vi "Measurement Logic.vi"() -> ()   [LabVIEW 2024, in "OneShot-PureTone.lvlib"]
uses:
  OneShot-PureTone.lvlib
  <vilib>/Plug-In SDKs/Measurements/Measure Call Context/Measure Call Context.lvclass
  Measurement Configuration.ctl
  Measurement Results.ctl
  <vilib>/DAQmx/read.llb/DAQmx Read (Analog Wfm 1Chan NSamp).vi
  <vilib>/DAQmx/create/channels.llb/DAQmx Create Channel (AI-Voltage-Basic).vi
  <vilib>/DAQmx/configure/timing.llb/DAQmx Timing (Sample Clock).vi
  <vilib>/DAQmx/create/channels.llb/DAQmx Create Channel (AO-FuncGen).vi
  <vilib>/DAQmx/miscellaneous.llb/DAQmx Fill In Error Info.vi
  <extravilib>/ChannelInstances/Event Messenger-bool/Instantiate.vi
  <resource>/objmgr/daqmx.rc
panel:
  out "measurement results":T1={"band start (Hz) out"=0.0, "band stop (Hz) out"=0.0, "detected frequency (Hz)"=0.0, "detected amplitude"=0.0, "acquired response"=[0.0], "measurement subset"=[0.0], "acquired response t0"=0.0, "acquired response dt"=0.0, "measurement subset t0"=0.0, "measurement subset dt"=0.0, "THD maximum harmonic out"=9} {"THD maximum harmonic out" min=-1 max=1000; "detected amplitude" format="%.3g"; "band stop (Hz) out" format="%.2f"; "band start (Hz) out" format="%.2f"}
  in  "measurement configuration":T2={"THD maximum harmonic"=1, "measurement duration (s)"=1.2, "measurement cycles"=32.0, "band start (Hz)"=32.0, "band stop (Hz)"=64.0, "settle time (s)"=-32.0, "settle cycles"=-64.0, "AI range"=-64.0, "output channel"="Dev1/ao0", "input channel"="Dev1/ai0", "frequency (Hz)"=1.0, "amplitude"=1.0, "sample rate (Hz)"=0.05} {"sample rate (Hz)" min=0.0 format="%.2p"; "amplitude" format="%.3g"; "frequency (Hz)" format="±  %.3g"; "settle cycles" min=0.0 format="%.2p"; "band stop (Hz)" format="%.2f"; "measurement cycles" min=1.0; "THD maximum harmonic" min=-1 max=1000}
  out "measure call context out":refnum<class "Measure Call Context.lvclass">
  in  "measure call context in":refnum<class "Measure Call Context.lvclass">
  out "error out":errorcluster
  in  "error in":errorcluster
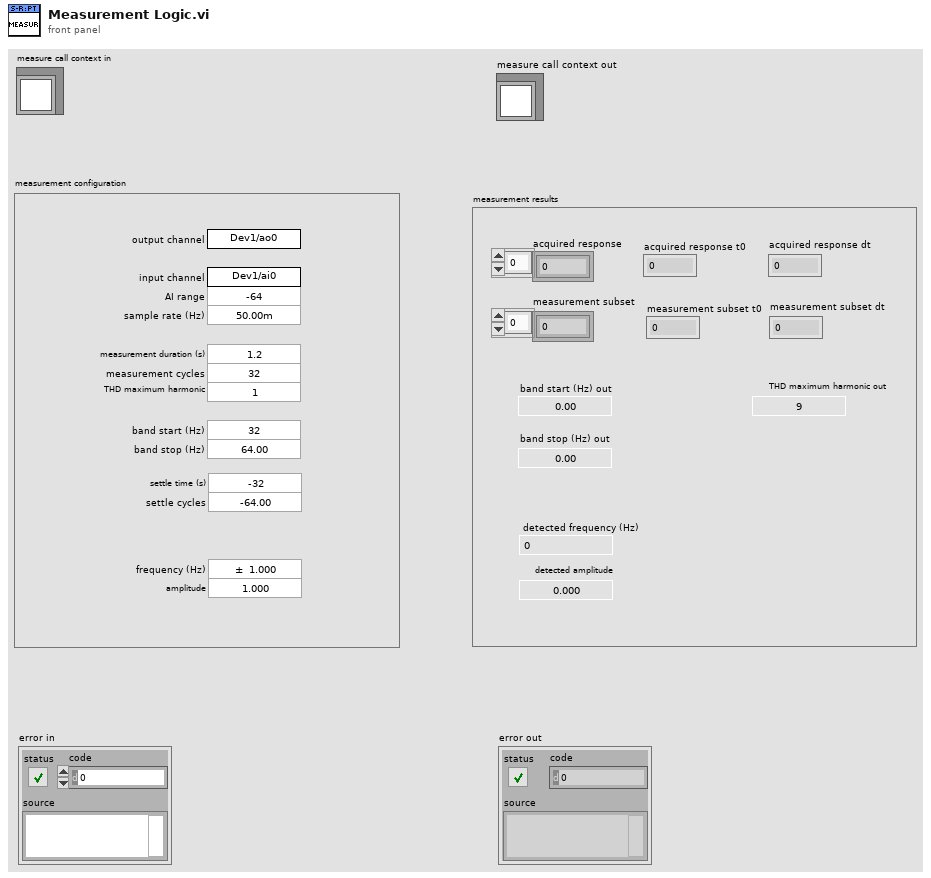
[diagram p1: front panel]
types:
  T1 = typedef "OneShot-PureTone.lvlib/Measurement Results.ctl" = cluster{"band start (Hz) out":dbl, "band stop (Hz) out":dbl, "detected frequency (Hz)":dbl, "detected amplitude":dbl, "acquired response":dbl[], "measurement subset":dbl[], "acquired response t0":dbl, "acquired response dt":dbl, "measurement subset t0":dbl, "measurement subset dt":dbl, "THD maximum harmonic out":i32}
  T2 = typedef "OneShot-PureTone.lvlib/Measurement Configuration.ctl" = cluster{"THD maximum harmonic":i32, "measurement duration (s)":dbl, "measurement cycles":dbl, "band start (Hz)":dbl, "band stop (Hz)":dbl, "settle time (s)":dbl, "settle cycles":dbl, "AI range":dbl, "output channel":string, "input channel":string, "frequency (Hz)":dbl, "amplitude":dbl, "sample rate (Hz)":dbl}
  T3 = typedef "Event Messenger-bool.lvlib/))Channel.ctl" = refnum<queue>
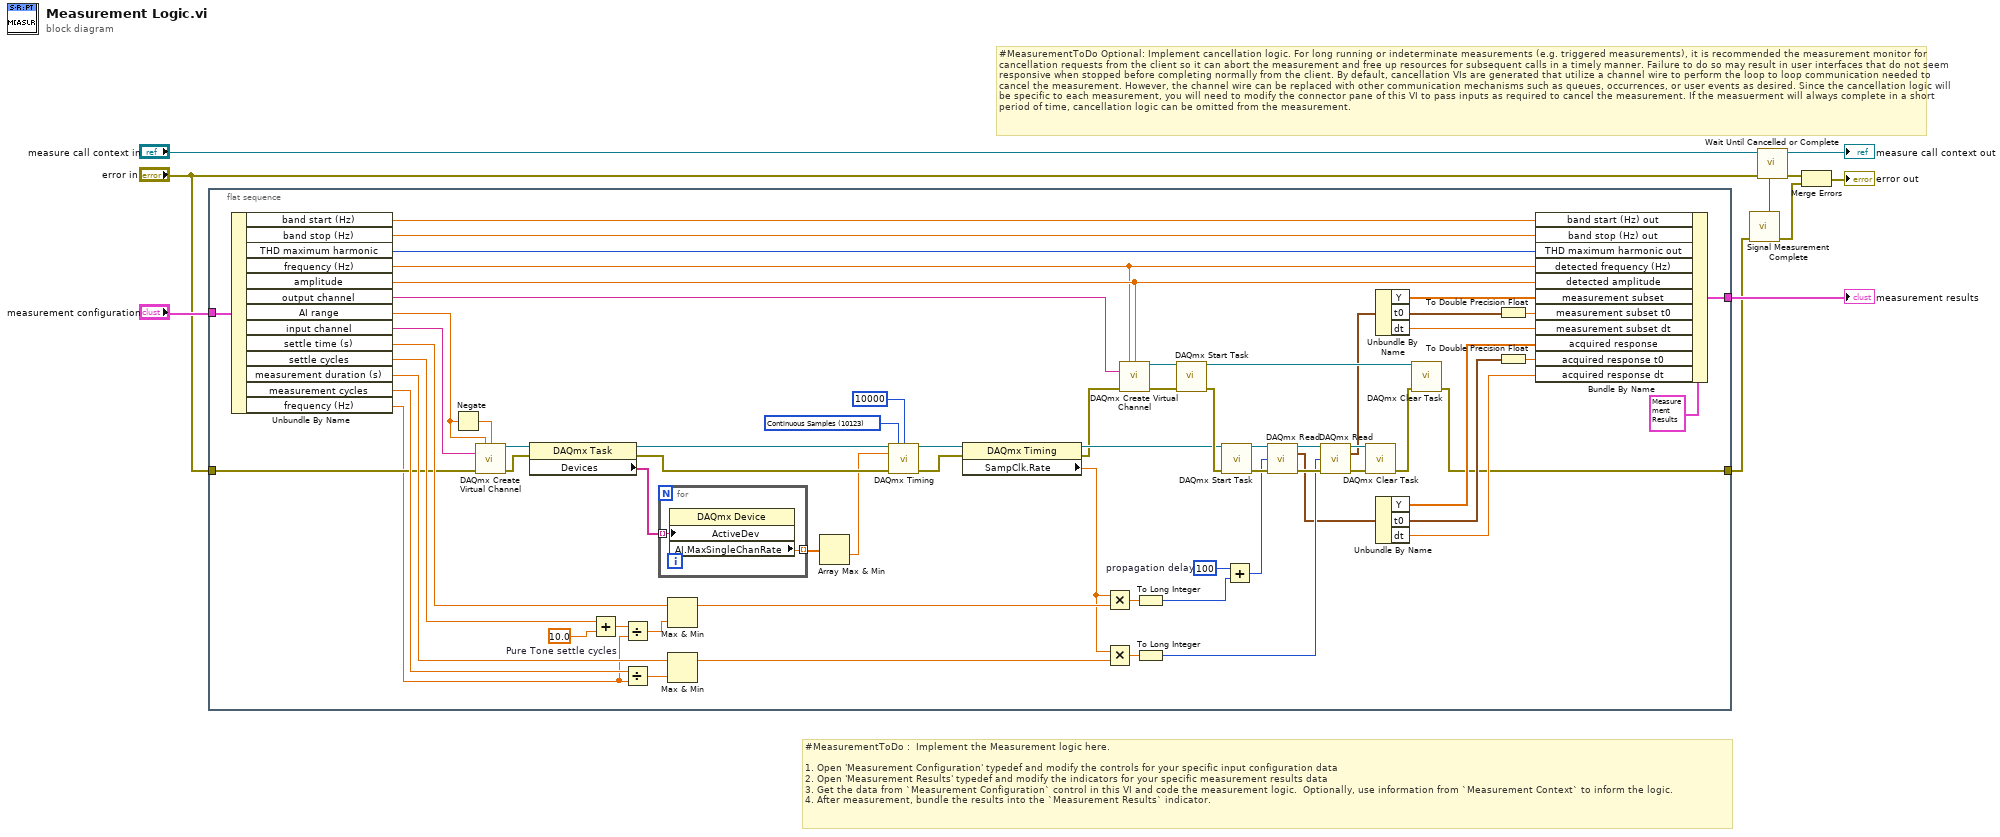
[diagram p0: block diagram]
diagram:
  # "#MeasurementToDo Optional: Implement cancellation logic. For long running or indeterminate measurements (e.g. triggered measurements), it is recommended the measurement monitor for cancellation requests from the client so it can abort the measurement and free up resources for subsequent calls in a timely manner. Failure to do so may result in user interfaces that do not seem responsive when stopped before completing normally from the client. By default, cancellation VIs are generated that utilize a channel wire to perform the loop to loop communication needed to cancel the measurement. However, the channel wire can be replaced with other communication mechanisms such as queues, occurrences, or user events as desired. Since the cancellation logic will be specific to each measurement, you will need to modify the connector pane of this VI to pass inputs as required to cancel the measurement. If the measuerment will always complete in a short period of time, cancellation logic can be omitted from the measurement."
  # "#MeasurementToDo :  Implement the Measurement logic here.\n\n1. Open 'Measurement Configuration' typedef and modify the controls for your specific input configuration data\n2. Open 'Measurement Results' typedef and modify the indicators for your specific measurement results data\n3. Get the data from `Measurement Configuration` control in this VI and code the measurement logic.  Optionally, use information from `Measurement Context` to inform the logic.\n4. After measurement, bundle the results into the `Measurement Results` indicator."
  n1 = flat-sequence {
    tunnel: "measurement configuration" -> [w74]
    tunnel: [w75] -> w9
    tunnel: "error in" -> [w20]
    tunnel: [w11] -> w5
    frame #0 {
      w27 = 10.0  # Pure Tone settle cycles
      w31 = 100  # propagation delay
      w62 = 10123 items=["Finite Samples"=10178, "Continuous Samples"=10123] ("sample mode")
      n2 = Unbundle By Name(w74) -> ("band start (Hz)"=w73:dbl, "band stop (Hz)"=w72:dbl, "THD maximum harmonic"=w71:i32, "frequency (Hz)"=w15:dbl, "amplitude"=w16:dbl, "output channel"=w19:string, "AI range"=w18:dbl, "input channel"=w17:string, "settle time (s)"=w25:dbl, "settle cycles"=w26:dbl, "measurement duration (s)"=w24:dbl, "measurement cycles"=w23:dbl, "frequency (Hz)"=w14:dbl)
      n3 = Negate(x=w18) -> (-x=w61:dbl)
      n4 = call-poly <vilib>:"DAQmx Create Virtual Channel.vi"("maximum value"=w18, "minimum value"=w61, "physical channels"=w17, "error in"=w20) -> ("task out"=w57:refnum<k21>, "error out"=w56:errorcluster)  [unwired: 10 in]
      n5 = property on="Property Node" class="DAQmx Task"(reference=w57, error in=w56) -> (reference out=w55:refnum<k21>, error out=w54:errorcluster, "Devices"=w53:tag[])
      n6 = Add(x=w26, y=w27) -> (x+y=w47:dbl)
      n7 = Divide(x=w47, y=w14) -> (x/y=w59:dbl)
      n8 = Divide(x=w23, y=w14) -> (x/y=w60:dbl)
      n9 = for {
        tunnel: w53 -> [w78] mode=indexing
        tunnel: [w77] -> w52 mode=indexing
        n10 = property on="Property Node" class="DAQmx Device"("ActiveDev"=w78) -> ("AI.MaxSingleChanRate"=w77:dbl)  [unwired: 2 in, 2 out]
      }
      n11 = Max & Min(x=w25, y=w59) -> (max(x,y)=w43:dbl)  [unwired: 1 out]
      n12 = Max & Min(x=w24, y=w60) -> (max(x,y)=w40:dbl)  [unwired: 1 out]
      n13 = Array Max & Min(array=w52) -> (min value=w28:dbl)  [unwired: 3 out]
      n14 = call-poly <vilib>:"DAQmx Timing.vi"("task/channels in"=w55, "sample mode"=w62, "samples per channel"=10000, "rate"=w28, "error in"=w54) -> ("task out"=w46:refnum<k21>, "error out"=w45:errorcluster)  [unwired: 9 in]
      n15 = property on="Property Node" class="DAQmx Timing"(reference=w46, error in=w45) -> (reference out=w44:refnum<k21>, error out=w12:errorcluster, "SampClk.Rate"=w39:dbl)
      n16 = Multiply(x=w39, y=w43) -> (x*y=w42:dbl)
      n17 = Multiply(x=w39, y=w40) -> (x*y=w41:dbl)
      n18 = call-poly <vilib>:"DAQmx Create Virtual Channel.vi"("frequency"=w15, "amplitude"=w16, "physical channels"=w19, "error in"=w12) -> ("task out"=w51:refnum<k21>, "error out"=w13:errorcluster)  [unwired: 10 in]
      n19 = To Long Integer(number=w42) -> (32bit integer=w30:i32)
      n20 = To Long Integer(number=w41) -> (32bit integer=w36:i32)
      n21 = call <vilib>:"DAQmx Start Task.vi"("task/channels in"=w51, "error in"=w13) -> ("task out"=w32:refnum<k21>, "error out"=w49:errorcluster)  [unwired: 12 in]
      n22 = call <vilib>:"DAQmx Start Task.vi"("task/channels in"=w44, "error in"=w49) -> ("task out"=w48:refnum<k21>, "error out"=w50:errorcluster)  [unwired: 12 in]
      n23 = Add(x=w31, y=w30) -> (x+y=w29:i32)
      n24 = call-poly <vilib>:"DAQmx Read.vi"("task/channels in"=w48, "number of samples per channel"=w29, "error in"=w50) -> ("task out"=w37:refnum<k21>, "data"=w21:waveform(dbl), "error out"=w38:errorcluster)  [unwired: 10 in]
      n25 = call-poly <vilib>:"DAQmx Read.vi"("task/channels in"=w37, "number of samples per channel"=w36, "error in"=w38) -> ("task out"=w34:refnum<k21>, "data"=w22:waveform(dbl), "error out"=w35:errorcluster)  [unwired: 10 in]
      n26 = call <vilib>:"DAQmx Clear Task.vi"("task in"=w34, "error in"=w35) -> ("error out"=w33:errorcluster)  [unwired: 13 in]
      n27 = Unbundle By Name(w22) -> ("Y"=w70:dbl[], "t0"=w69:timestamp, "dt"=w67:dbl)
      n28 = Unbundle By Name(w21) -> ("Y"=w66:dbl[], "t0"=w64:timestamp, "dt"=w65:dbl)
      n29 = call <vilib>:"DAQmx Clear Task.vi"("task in"=w32, "error in"=w33) -> ("error out"=w11:errorcluster)  [unwired: 13 in]
      n30 = To Double Precision Float(number=w69) -> (double precision float=w68:dbl)
      n31 = To Double Precision Float(number=w64) -> (double precision float=w63:dbl)
      n32 = Bundle By Name(cluster=T1 {"band start (Hz) out"=0.0, "band stop (Hz) out"=0.0, "detected frequency (Hz)"=0.0, "detected amplitude"=0.0, "acquired response"=[], "measurement subset"=[], "acquired response t0"=0.0, "acquired response dt"=0.0, "measurement subset t0"=0.0, "measurement subset dt"=0.0, "THD maximum harmonic out"=9} ("Measurement Results"), "band start (Hz) out"=w73, "band stop (Hz) out"=w72, "THD maximum harmonic out"=w71, "detected frequency (Hz)"=w15, "detected amplitude"=w16, "measurement subset"=w70, "measurement subset t0"=w68, "measurement subset dt"=w67, "acquired response"=w66, "acquired response t0"=w63, "acquired response dt"=w65) -> (w75:T1)
    }
  }
  n33 = call "Signal Measurement Complete.vi"("error in (no error)"=w5) -> ("error out"=w3:errorcluster, "done channel"=w4:T3)  [unwired: 9 in]
  n34 = call "Wait Until Cancelled or Complete.vi"("done channel"=w4, "error in (no error)"="error in", "measure call context in"="measure call context in") -> ("error out"=w2:errorcluster, "measure call context out"=→"measure call context out":refnum<class "Measure Call Context.lvclass">)  [unwired: 7 in]
  n35 = Merge Errors(w2, w3) -> (→"error out":errorcluster)
  "measurement results" <- w9
